vi "Motors Open.vi"(2 "error in (no error)":errorcluster, 3 "VISA in":refnum<visa-resource-name>="COM7") -> (0 "error out":errorcluster, 1 "VISA out":refnum<visa-resource-name>)   [LabVIEW 2018]
uses:
  <vilib>/Instr/_visa.llb/VISA Configure Serial Port (Instr).vi
panel:
  in  "Wait after configuring channel, but before communicating":u32=100
  in  "Eanble 4":bool=TRUE
  in  "Enable 3":bool=TRUE
  in  "Enable 2":bool=TRUE
  in  "Enable 1":bool=TRUE
  out "read buffer 4":string
  out "read buffer 3":string
  out "read buffer 2":string
  out "read buffer 1":string
  in  "Initial command 4":string="4ID"
  in  "Initial command 3":string="3ID"
  in  "Initial command 2":string="2ID"
  in  "Initial command 1":string="1ID"
  in  "Data Bits":i32=7
  in  "flow control":u16(ring) items=["None", "XON/XOFF", "RTS/CTS", "XON/XOFF & RTS/CTS", "DTR/DSR", "XON/XOFF & DTR/DSR"]
  in  "baud rate":u32=9600
  in  "timeout (ms)":u32=1000
  in  "stop bits (10: 1 bit)":u16(ring)=10 items=["1.0"=10, "1.5"=15, "2.0"=20]
  in  "parity (0:none)":enum16{"None", "Odd", "Even", "Mark", "Space"}(ring)=enum."Even"
  in  "termination char\n(0xA = '\\n' = LF)":u8=10 format="%.0x"
  # "Motor Settings Indicated in the Manual:\nFlow Control: RTS/CTS\nTermination Char: A (CR/LF)\nBaud Rate: 9600\nData Bits: 7\nPairity: Even\nStop Bits: 1\n\nUsing no flow control works just as well."
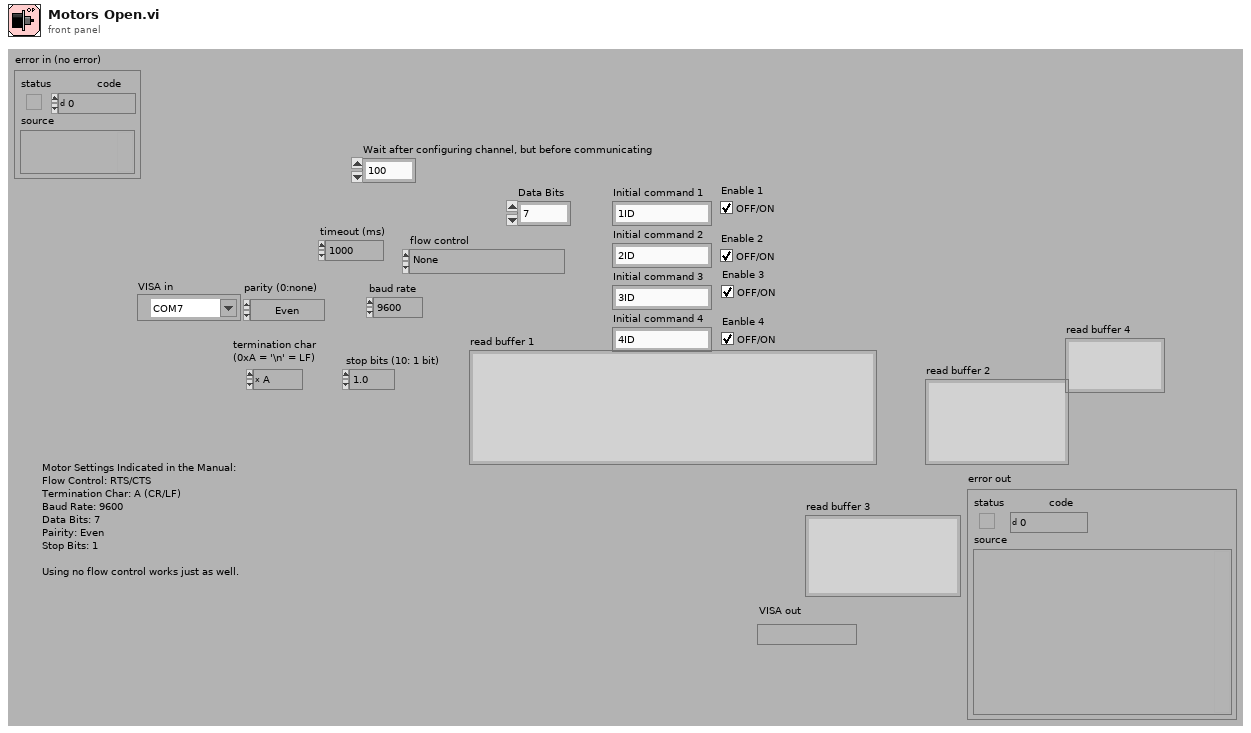
[diagram p1: front panel]
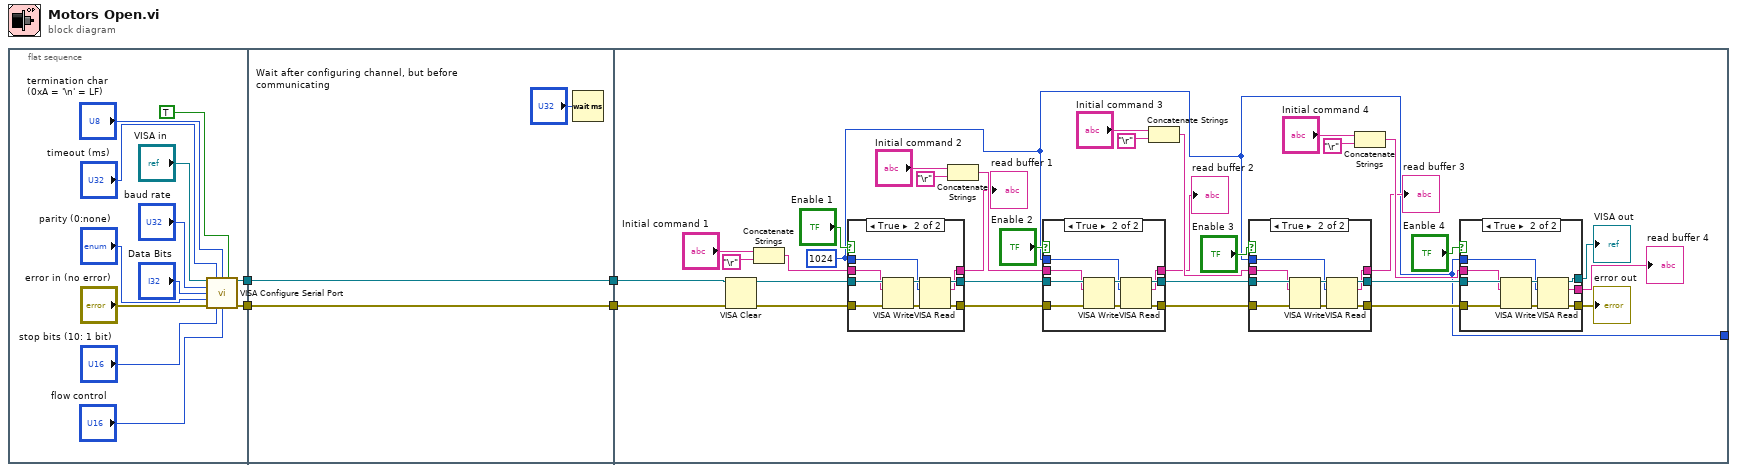
[diagram p0: block diagram]
diagram:
  n1 = flat-sequence {
    tunnel: [w7] -> w4
    tunnel: [w6] -> w3
    tunnel: w4 -> [w19]
    tunnel: w3 -> [w18]
    tunnel: [w19] -> w2
    tunnel: [w18] -> w1
    tunnel: [w25] -> _
    tunnel: w2 -> [w23]
    tunnel: w1 -> [w21]
    frame #0 {
      n2 = call-poly "VISA Configure Serial Port"("VISA resource name"="VISA in", "timeout (10sec)"="timeout (ms)", "termination char\n(0xA = '\\n' = LF)"="termination char\n(0xA = '\\n' = LF)", "Enable Termination\nChar (T)"=TRUE, "baud rate (9600)"="baud rate", "data bits (8)"="Data Bits", "parity (0:none)"="parity (0:none)", "error in (no error)"="error in (no error)", "stop bits (10: 1 bit)"="stop bits (10: 1 bit)", "flow control (0:none)"="flow control") -> ("VISA resource name out"=w7:refnum<visa-resource-name>, "error out"=w6:errorcluster)  [unwired: 4 in]
    }
    frame #1 {
      n3 = Wait (ms)(milliseconds to wait="Wait after configuring channel, but before communicating") -> ()  [unwired: 1 out]
    }
    frame #2 {
      w25 = u32 1024 ("byte count")
      n4 = VISA Clear(VISA resource name=w23, error in (no error)=w21) -> (VISA resource name out=w22:refnum<visa-resource-name>, error out=w20:errorcluster)
      n5 = Concatenate Strings("Initial command 1", "\r") -> (w26:string)
      n6 = case shown="True" "Enable 1" {
        tunnel: w22 -> [w87 w95]
        tunnel: [w87 w93] -> w34
        tunnel: w20 -> [w86 w92]
        tunnel: [w86 w91] -> w35
        tunnel: w25 -> [_ w90]
        tunnel: [_ w89] -> w36
        tunnel: w26 -> [_ w88]
        frame False {
        }
        frame True {
          n7 = VISA Write(VISA resource name=w95, write buffer=w88, error in (no error)=w92) -> (VISA resource name out=w94:refnum<visa-resource-name>, error out=w96:errorcluster)  [unwired: 1 out]
          n8 = VISA Read(VISA resource name=w94, byte count=w90, error in (no error)=w96) -> (VISA resource name out=w93:refnum<visa-resource-name>, read buffer=w89:string, error out=w91:errorcluster)  [unwired: 1 out]
        }
      }
      "read buffer 1" <- w36
      n9 = Concatenate Strings("Initial command 2", "\r") -> (w38:string)
      n10 = case shown="True" "Enable 2" {
        tunnel: w34 -> [w76 w84]
        tunnel: w35 -> [w75 w81]
        tunnel: [w76 w82] -> w39
        tunnel: [w75 w80] -> w40
        tunnel: w25 -> [_ w79]
        tunnel: [_ w78] -> w37
        tunnel: w38 -> [_ w77]
        frame False {
        }
        frame True {
          n11 = VISA Write(VISA resource name=w84, write buffer=w77, error in (no error)=w81) -> (VISA resource name out=w83:refnum<visa-resource-name>, error out=w85:errorcluster)  [unwired: 1 out]
          n12 = VISA Read(VISA resource name=w83, byte count=w79, error in (no error)=w85) -> (VISA resource name out=w82:refnum<visa-resource-name>, read buffer=w78:string, error out=w80:errorcluster)  [unwired: 1 out]
        }
      }
      "read buffer 2" <- w37
      n13 = Concatenate Strings("Initial command 3", "\r") -> (w42:string)
      n14 = case shown="True" "Enable 3" {
        tunnel: w39 -> [w65 w73]
        tunnel: [w65 w71] -> w43
        tunnel: w40 -> [w64 w70]
        tunnel: [w64 w69] -> w44
        tunnel: w25 -> [_ w68]
        tunnel: [_ w67] -> w41
        tunnel: w42 -> [_ w66]
        frame False {
        }
        frame True {
          n15 = VISA Write(VISA resource name=w73, write buffer=w66, error in (no error)=w70) -> (VISA resource name out=w72:refnum<visa-resource-name>, error out=w74:errorcluster)  [unwired: 1 out]
          n16 = VISA Read(VISA resource name=w72, byte count=w68, error in (no error)=w74) -> (VISA resource name out=w71:refnum<visa-resource-name>, read buffer=w67:string, error out=w69:errorcluster)  [unwired: 1 out]
        }
      }
      "read buffer 3" <- w41
      n17 = Concatenate Strings("Initial command 4", "\r") -> (w48:string)
      n18 = case shown="True" "Eanble 4" {
        tunnel: w43 -> [w54 w62]
        tunnel: w44 -> [w53 w60]
        tunnel: [w54 w59] -> w45
        tunnel: [w53 w58] -> w46
        tunnel: [_ w57] -> w47
        tunnel: w48 -> [_ w56]
        tunnel: w25 -> [_ w55]
        frame False {
        }
        frame True {
          n19 = VISA Write(VISA resource name=w62, write buffer=w56, error in (no error)=w60) -> (VISA resource name out=w61:refnum<visa-resource-name>, error out=w63:errorcluster)  [unwired: 1 out]
          n20 = VISA Read(VISA resource name=w61, byte count=w55, error in (no error)=w63) -> (VISA resource name out=w59:refnum<visa-resource-name>, read buffer=w57:string, error out=w58:errorcluster)  [unwired: 1 out]
        }
      }
      "error out" <- w46
      "VISA out" <- w45
      "read buffer 4" <- w47
    }
  }
